vi "Example (array).vi"() -> ()   [LabVIEW 2017]
uses:
  Example.ctl
  source/TreeLUT.lvclass
panel:
  in  "Copies":i32=5
  out "Attribute":string
  in  "Stop":bool
  out "Value":variant
  in  "CTD Tree":string(tree)
  in  "?":T1={"Numeric"={"I32"=0, "DBL"=0.0}, "Boolean"={"Boolean"=TRUE}, "String"={"String"="", "Path"=path ""}, "Timing"={"Time Stamp"=timestamp(0 s since 1904-01-01), "Waveform"={"t0"=timestamp(0 s since 1904-01-01), "dt"=1.0, "Y"=[]}}, "Objects & Variants"={"LabVIEW Object"=refnum, "Variant"=variant}, "Refnum"={"NAR"=refnum, "DigNum"=refnum, "queue"=refnum, "notifier"=refnum}}
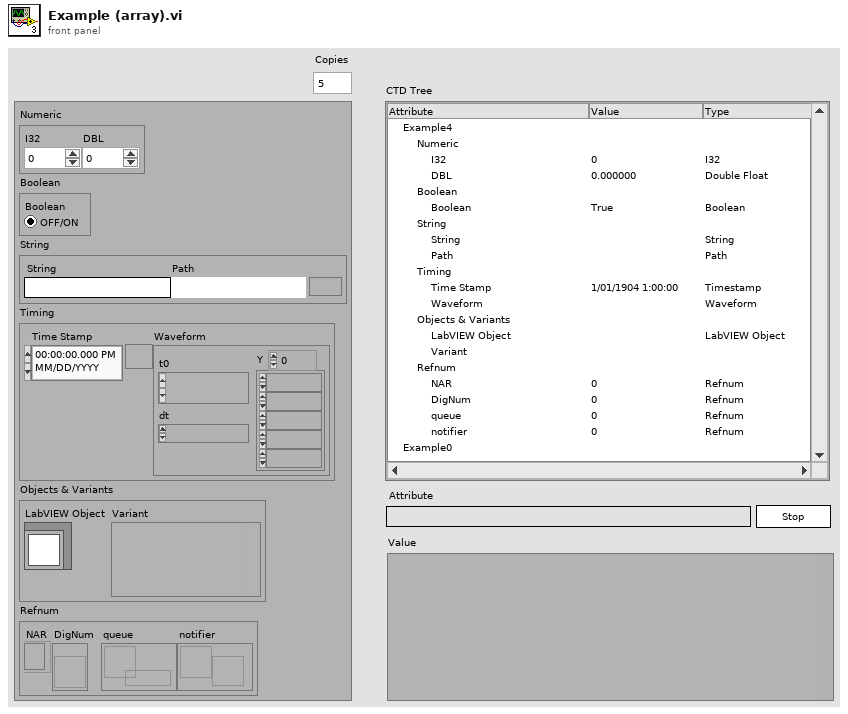
[diagram p1: front panel]
types:
  T1 = typedef "Example.ctl" = cluster{"Numeric":cluster{"I32":i32, "DBL":dbl}, "Boolean":cluster{"Boolean":bool}, "String":cluster{"String":string, "Path":path}, "Timing":cluster{"Time Stamp":timestamp, "Waveform":waveform(dbl)}, "Objects & Variants":cluster{"LabVIEW Object":refnum<class>, "Variant":variant}, "Refnum":cluster{"NAR":refnum<file>, "DigNum":refnum<vi>, "queue":refnum<queue>, "notifier":refnum<notifier>}}
  T2 = cluster{"Left Cell String":string, "Child Text":string[], "Child Tag":string, "Item Indent":i32, "Child Only?":bool, "Glyph Index":i32}[]
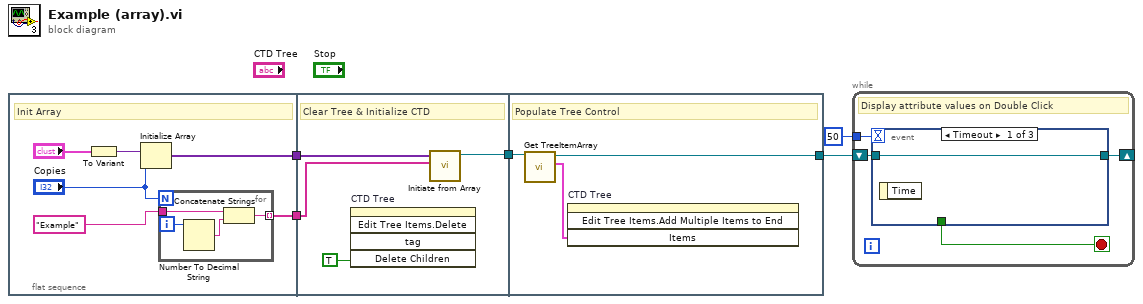
[diagram p0: block diagram]
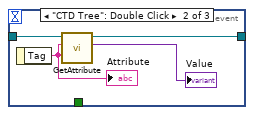
[diagram p2: hidden frame]
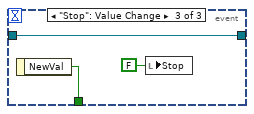
[diagram p3: hidden frame]
diagram:
  n1 = flat-sequence {
    tunnel: [w9] -> w2
    tunnel: [w6] -> w1
    tunnel: [w18] -> w5
    tunnel: w2 -> [w17]
    tunnel: w1 -> [w16]
    tunnel: w5 -> [w21]
    tunnel: [w20] -> w4
    frame #0 {
      # "Init Array"
      n2 = To Variant(anything="?") -> (Variant=w10:variant)
      n3 = Initialize Array(w10, "Copies") -> (w9:variant[])
      n4 = for {
        N: "Copies" -> [_]
        tunnel: "Example" -> [w13]
        tunnel: [w12] -> w6 mode=indexing
        i -> [w15]
        n5 = Number To Decimal String(number=w15) -> (decimal integer string=w14:string)  [unwired: 1 in]
        n6 = Concatenate Strings(w13, w14) -> (w12:string)
      }
    }
    frame #1 {
      # "Clear Tree & Initialize CTD"
      n7 = invoke on="CTD Tree" class="Tree (strict)" method="Edit Tree Items.Delete"("Delete Children"=TRUE) -> ()  [unwired: 4 in, 5 out]
      n8 = call "Initiate from Array.vi"("Prefix Array"=w16, "Array"=w17) -> ("ClusterTree out"=w18:refnum<class "TreeLUT.lvclass">)  [unwired: 8 in, 1 out]
    }
    frame #2 {
      # "Populate Tree Control"
      n9 = call "Get TreeItemArray.vi"("ClusterTree in"=w21) -> ("TreeItem Array"=w22:T2, "ClusterTree out"=w20:refnum<class "TreeLUT.lvclass">)  [unwired: 8 in, 1 out]
      n10 = invoke on="CTD Tree" class="Tree (strict)" method="Edit Tree Items.Add Multiple Items to End"("Items"=w22) -> ()  [unwired: 3 in, 4 out]
    }
  }
  n11 = while {
    shift-right: [w25] -> _
    shift-left: w4 -> [w26]
    tunnel: 50 -> [w24]
    stop <- w23 stop-if-true
    # "Display attribute values on Double Click"
    n12 = event shown="[0] Timeout" {
      selector: _ -> [_ _ _]
      dyn-events: _ -> [_ _ _]
      timeout: w24 -> [_ _ _]
      tunnel: w26 -> [w27 w30 w33]
      tunnel: [w27 w29 w33] -> w25
      tunnel: [_ _ w34] -> w23
      event Timeout {
        n13 = event-data() -> ()  [unwired: 1 in, 1 out]
      }
      event "CTD Tree": Double Click {
        n14 = event-data() -> ("Tag"=w28:string)  [unwired: 1 in]
        "Attribute" <- w28
        n15 = call "GetAttribute.vi"("Attribute"=w28, "ClusterTreeDict in"=w30) -> ("Value"=→"Value":variant, "ClusterTreeDict out"=w29:refnum<class "TreeLUT.lvclass">)  [unwired: 7 in, 1 out]
      }
      event "Stop": Value Change {
        n16 = event-data() -> ("NewVal"=w34:bool)  [unwired: 1 in]
        n17 = local write "Stop"(FALSE ("Stop")) -> ()
      }
    }
  }
